vi "RTS Extract Door Test Array.vi"(8 "error in (no error)":errorcluster, 9 "Section Name":string, 10 "section names":string[](array[string]), 11 "Refnum in":T4) -> (0 "error out":errorcluster, 2 "Array":T1[](array[typedef]) {"Start Time" format="%<%X\n%x>T"; "End Time" format="%<%X\n%x>T"}, 3 "Refnum out":T4, 4 "key names":string[][](array[string]))   [LabVIEW 2016]
uses:
  Type Definitions/RTS Door Ops Client.ctl
  Type Definitions/RTS Door Opening Schedule.ctl
  Type Definitions/RTS Door Ops Sequence.ctl
  <vilib>/Utility/config.llb/Config Data RefNum.ctl
  <vilib>/Utility/config.llb/Read Key (Double).vi
  <vilib>/Utility/config.llb/Read Key (Boolean).vi
  <vilib>/Utility/config.llb/Read Key (U32).vi
  <vilib>/Utility/config.llb/NI_LVConfig.lvlib
panel:
  out "Array 2":T1[](array[typedef]) {"Start Time" format="%<%X\n%x>T"; "End Time" format="%<%X\n%x>T"}
  # "Chamber Conditions:"
  # "Chamber Conditions:"
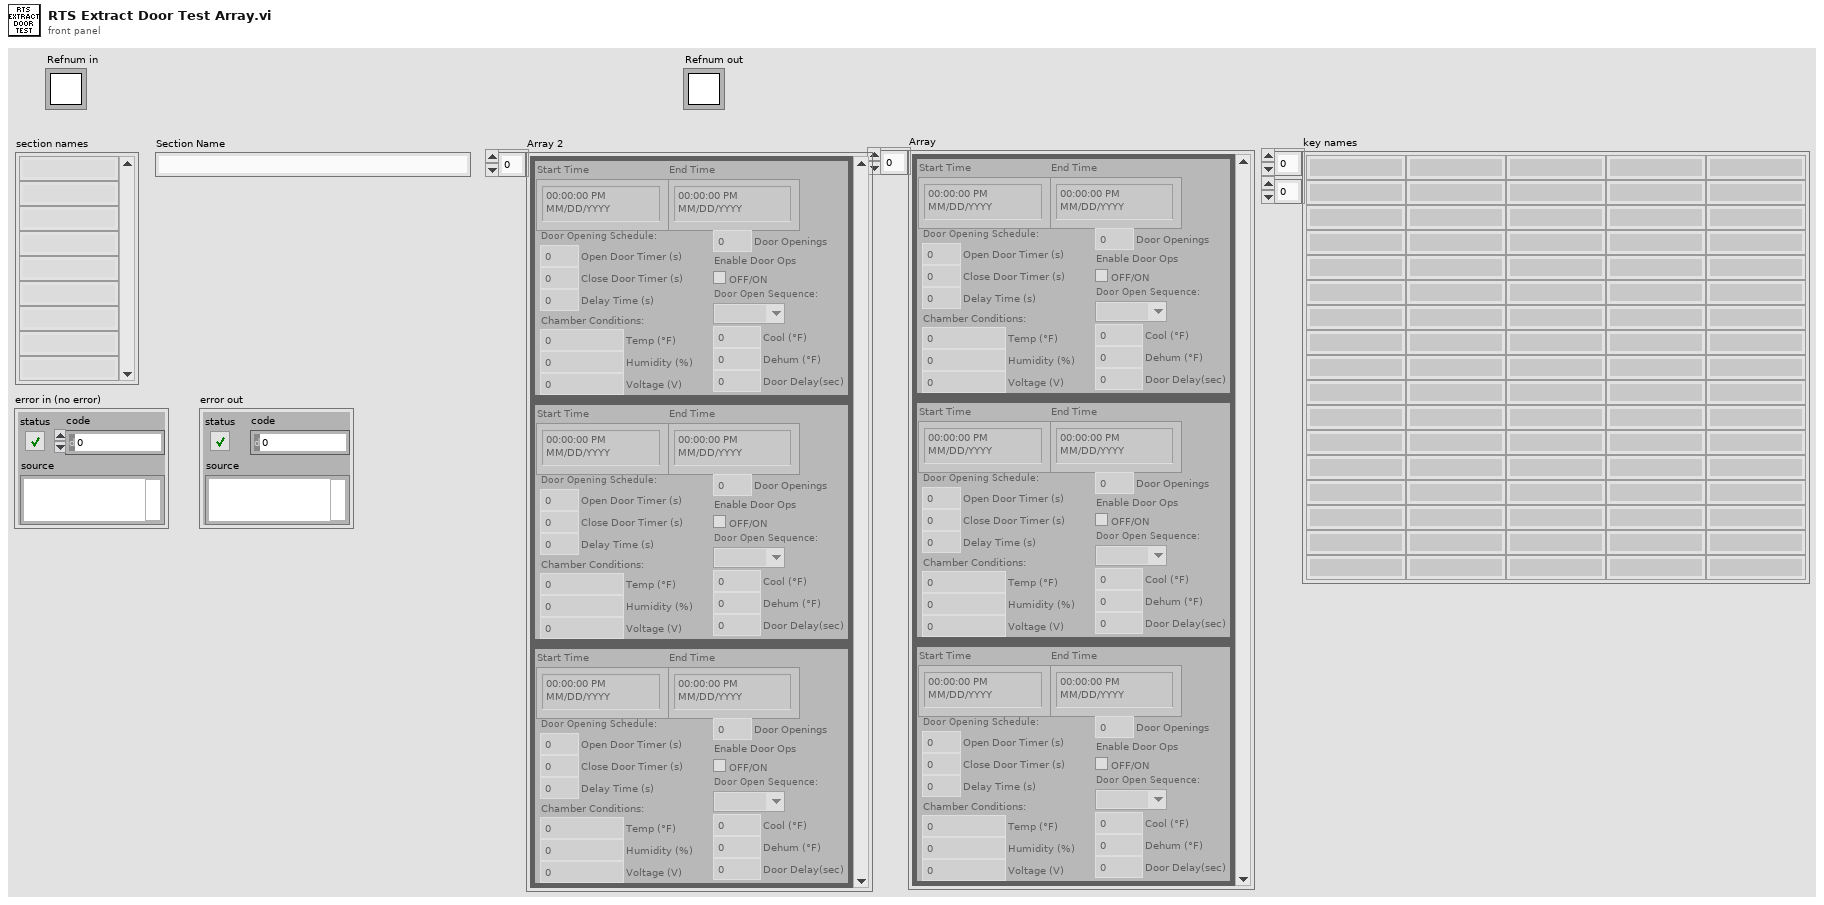
[diagram p1: front panel]
types:
  T1 = typedef "RTS Door Ops Client.ctl" = cluster{"End Time":timestamp, "Start Time":timestamp, "Door Opening Schedule:":T2, "Enable Door Ops":bool, "Door Openings":u32, "Temp (°F)":dbl, "Humidity (%)":dbl, "Voltage (V)":dbl, "Door Open Sequence:":T3, "Door Delay(sec)":dbl, "Dehum (°F)":dbl, "Cool (°F)":dbl}
  T2 = typedef "RTS Door Opening Schedule.ctl" = cluster{"Open Door Timer (s)":dbl, "Delay Time (s)":dbl, "Close Door Timer (s)":dbl}
  T3 = typedef "RTS Door Ops Sequence.ctl" = enum16{"", "1st", "2nd", "3rd"}
  T4 = typedef "NI_LVConfig.lvlib/Config Data RefNum.ctl" = refnum<k1>
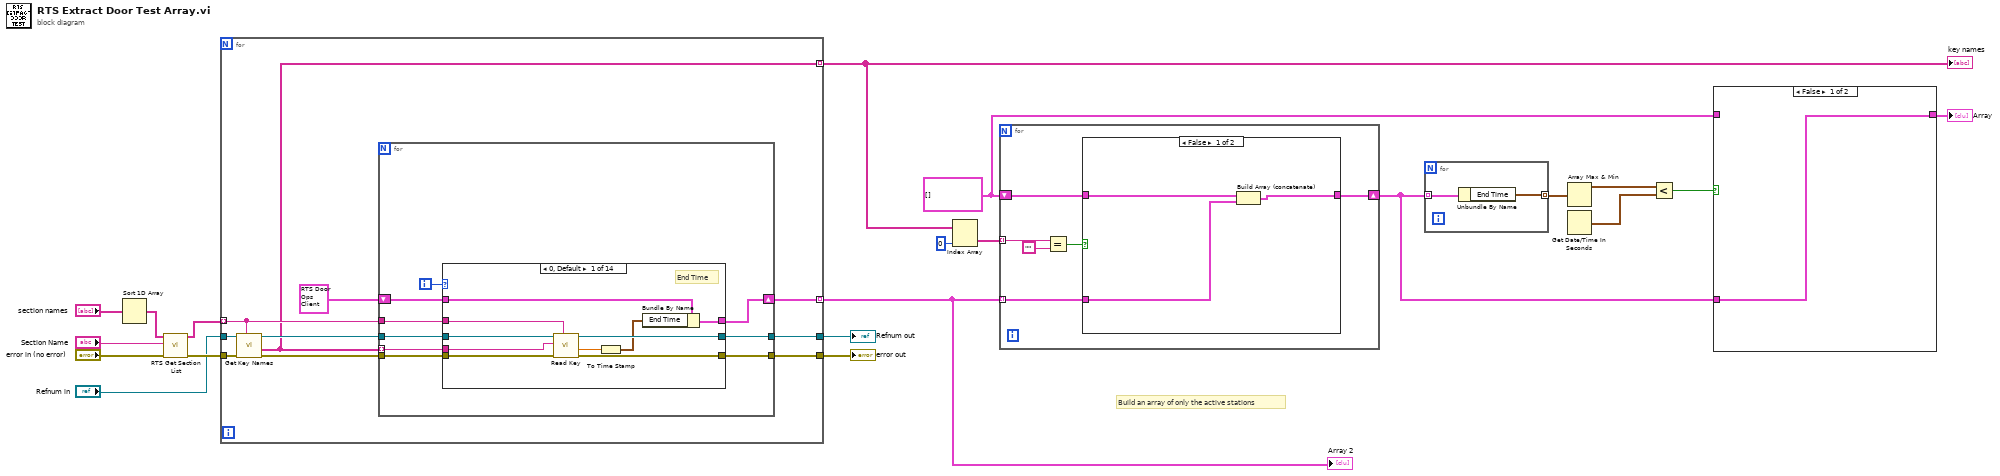
[diagram p0: block diagram]
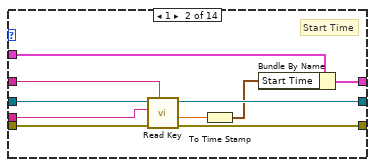
[diagram p4: hidden frame]
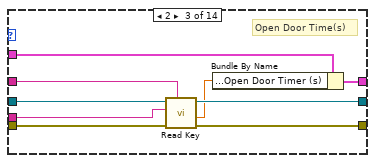
[diagram p5: hidden frame]
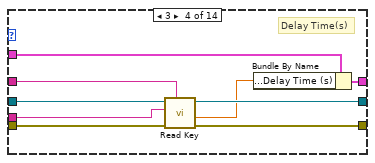
[diagram p6: hidden frame]
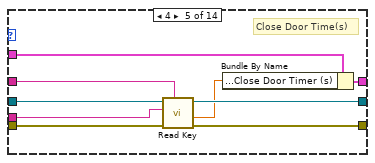
[diagram p7: hidden frame]
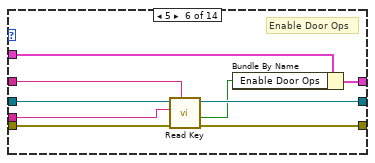
[diagram p8: hidden frame]
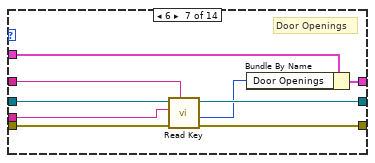
[diagram p9: hidden frame]
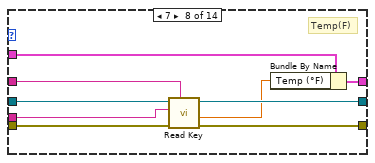
[diagram p10: hidden frame]
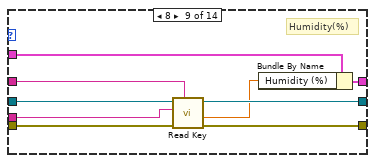
[diagram p11: hidden frame]
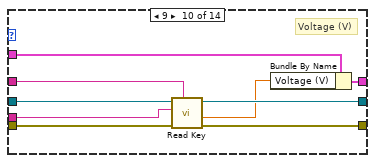
[diagram p12: hidden frame]
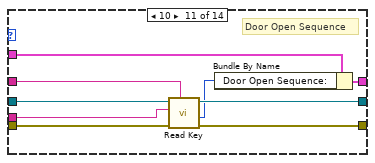
[diagram p13: hidden frame]
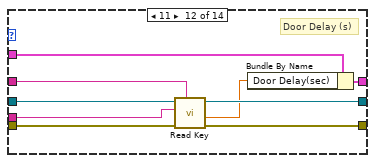
[diagram p14: hidden frame]
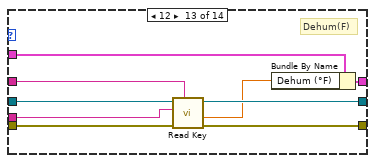
[diagram p15: hidden frame]
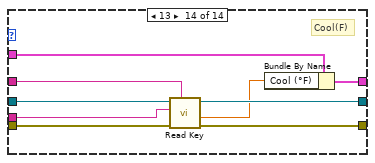
[diagram p16: hidden frame]
diagram:
  w3 = T1[] []
  # "Build an array of only the active stations"
  n1 = Sort 1D Array(array="section names") -> (sorted array=w14:string[])
  n2 = call "RTS Get Section List.vi"("Error In"="error in (no error)", "Section Name"="Section Name", "Sorted Array"=w14) -> ("Error Out"=w20:errorcluster, "Parsed Array"=w17:string[])  [unwired: 7 in]
  n3 = for {
    tunnel: w17 -> [w24] mode=indexing
    tunnel: [w30] -> w8 mode=indexing
    tunnel: "Refnum in" -> [w29]
    tunnel: [w23] -> w15
    tunnel: w20 -> [w28]
    tunnel: [w22] -> w16
    tunnel: [w21] -> w11 mode=indexing
    n4 = call <vilib>:"Get Key Names.vi"("section"=w24, "error in (no error)"=w28, "refnum"=w29) -> ("error out"=w27:errorcluster, "key names"=w21:string[], "refnum out"=w26:T4)  [unwired: 5 in, 1 out]
    n5 = for {
      tunnel: w21 -> [w35] mode=indexing
      shift-right: [w33] -> w30
      shift-left: T1 {"End Time"=timestamp(0 s since 1904-01-01), "Start Time"=timestamp(0 s since 1904-01-01), "Door Opening Schedule:"={"Open Door Timer (s)"=0.0, "Delay Time (s)"=0.0, "Close Door Timer (s)"=0.0}, "Enable Door Ops"=FALSE, "Door Openings"=0, "Temp (°F)"=0.0, "Humidity (%)"=0.0, "Voltage (V)"=0.0, "Door Open Sequence:"=enum."", "Door Delay(sec)"=0.0, "Dehum (°F)"=0.0, "Cool (°F)"=0.0} ("element") -> [w34]
      tunnel: w24 -> [w32]
      tunnel: w26 -> [w36]
      tunnel: [w37] -> w23
      tunnel: w27 -> [w39]
      tunnel: [w38] -> w22
      i -> [w31]
      n6 = case shown="0, Default" w31 {
        tunnel: w39 -> [w48 w58 w68 w76 w86 w94 w103 w112 w121 w130 w139 w148 w157 w167]
        tunnel: [w46 w57 w67 w75 w85 w93 w102 w111 w120 w129 w138 w147 w156 w166] -> w38
        tunnel: [w47 w56 w66 w74 w83 w92 w101 w110 w119 w128 w137 w146 w155 w165] -> w37
        tunnel: w36 -> [w49 w59 w65 w77 w84 w95 w104 w113 w122 w131 w140 w149 w158 w164]
        tunnel: w35 -> [w45 w54 w63 w72 w81 w90 w99 w108 w117 w126 w135 w144 w154 w162]
        tunnel: w34 -> [w43 w52 w62 w71 w80 w89 w98 w107 w116 w125 w134 w143 w152 w161]
        tunnel: [w42 w51 w61 w70 w79 w88 w97 w106 w115 w124 w133 w142 w151 w160] -> w33
        tunnel: w32 -> [w44 w55 w64 w73 w82 w91 w100 w109 w118 w127 w136 w145 w153 w163]
        frame 0, Default {
          # "End Time"
          n7 = call-poly <vilib>:"Read Key.vi"("section"=w44, "error in (no error)"=w48, "key"=w45, "refnum"=w49) -> ("error out"=w46:errorcluster, "value"=w41:dbl, "refnum out"=w47:T4)  [unwired: 4 in, 1 out]
          n8 = To Time Stamp(1:w41) -> (0:w40:timestamp)
          n9 = Bundle By Name(cluster=w43, "End Time"=w40) -> (w42:T1)
        }
        frame 1 {
          # "Start Time"
          n10 = call-poly <vilib>:"Read Key.vi"("section"=w55, "error in (no error)"=w58, "key"=w54, "refnum"=w59) -> ("error out"=w57:errorcluster, "value"=w53:dbl, "refnum out"=w56:T4)  [unwired: 4 in, 1 out]
          n11 = To Time Stamp(1:w53) -> (0:w50:timestamp)
          n12 = Bundle By Name(cluster=w52, "Start Time"=w50) -> (w51:T1)
        }
        frame 2 {
          # "Open Door Time(s)"
          n13 = call-poly <vilib>:"Read Key.vi"("section"=w64, "error in (no error)"=w68, "key"=w63, "refnum"=w65) -> ("error out"=w67:errorcluster, "value"=w60:dbl, "refnum out"=w66:T4)  [unwired: 4 in, 1 out]
          n14 = Bundle By Name(cluster=w62, "Door Opening Schedule:.Open Door Timer (s)"=w60) -> (w61:T1)
        }
        frame 3 {
          # "Delay Time(s)"
          n15 = call-poly <vilib>:"Read Key.vi"("section"=w73, "error in (no error)"=w76, "key"=w72, "refnum"=w77) -> ("error out"=w75:errorcluster, "value"=w69:dbl, "refnum out"=w74:T4)  [unwired: 4 in, 1 out]
          n16 = Bundle By Name(cluster=w71, "Door Opening Schedule:.Delay Time (s)"=w69) -> (w70:T1)
        }
        frame 4 {
          # "Close Door Time(s)"
          n17 = call-poly <vilib>:"Read Key.vi"("section"=w82, "error in (no error)"=w86, "key"=w81, "refnum"=w84) -> ("error out"=w85:errorcluster, "value"=w78:dbl, "refnum out"=w83:T4)  [unwired: 4 in, 1 out]
          n18 = Bundle By Name(cluster=w80, "Door Opening Schedule:.Close Door Timer (s)"=w78) -> (w79:T1)
        }
        frame 5 {
          # "Enable Door Ops"
          n19 = call-poly <vilib>:"Read Key.vi"("section"=w91, "error in (no error)"=w94, "key"=w90, "refnum"=w95) -> ("error out"=w93:errorcluster, "value"=w87:bool, "refnum out"=w92:T4)  [unwired: 4 in, 1 out]
          n20 = Bundle By Name(cluster=w89, "Enable Door Ops"=w87) -> (w88:T1)
        }
        frame 6 {
          # "Door Openings"
          n21 = call-poly <vilib>:"Read Key.vi"("section"=w100, "error in (no error)"=w103, "key"=w99, "refnum"=w104) -> ("error out"=w102:errorcluster, "value"=w96:u32, "refnum out"=w101:T4)  [unwired: 4 in, 1 out]
          n22 = Bundle By Name(cluster=w98, "Door Openings"=w96) -> (w97:T1)
        }
        frame 7 {
          # "Temp(F)"
          n23 = call-poly <vilib>:"Read Key.vi"("section"=w109, "error in (no error)"=w112, "key"=w108, "refnum"=w113) -> ("error out"=w111:errorcluster, "value"=w105:dbl, "refnum out"=w110:T4)  [unwired: 4 in, 1 out]
          n24 = Bundle By Name(cluster=w107, "Temp (°F)"=w105) -> (w106:T1)
        }
        frame 8 {
          # "Humidity(%)"
          n25 = call-poly <vilib>:"Read Key.vi"("section"=w118, "error in (no error)"=w121, "key"=w117, "refnum"=w122) -> ("error out"=w120:errorcluster, "value"=w114:dbl, "refnum out"=w119:T4)  [unwired: 4 in, 1 out]
          n26 = Bundle By Name(cluster=w116, "Humidity (%)"=w114) -> (w115:T1)
        }
        frame 9 {
          # "Voltage (V)"
          n27 = call-poly <vilib>:"Read Key.vi"("section"=w127, "error in (no error)"=w130, "key"=w126, "refnum"=w131) -> ("error out"=w129:errorcluster, "value"=w123:dbl, "refnum out"=w128:T4)  [unwired: 4 in, 1 out]
          n28 = Bundle By Name(cluster=w125, "Voltage (V)"=w123) -> (w124:T1)
        }
        frame 10 {
          # "Door Open Sequence"
          n29 = call-poly <vilib>:"Read Key.vi"("section"=w136, "error in (no error)"=w139, "key"=w135, "refnum"=w140) -> ("error out"=w138:errorcluster, "value"=w132:u32, "refnum out"=w137:T4)  [unwired: 4 in, 1 out]
          n30 = Bundle By Name(cluster=w134, "Door Open Sequence:"=w132) -> (w133:T1)
        }
        frame 11 {
          # "Door Delay (s)"
          n31 = call-poly <vilib>:"Read Key.vi"("section"=w145, "error in (no error)"=w148, "key"=w144, "refnum"=w149) -> ("error out"=w147:errorcluster, "value"=w141:dbl, "refnum out"=w146:T4)  [unwired: 4 in, 1 out]
          n32 = Bundle By Name(cluster=w143, "Door Delay(sec)"=w141) -> (w142:T1)
        }
        frame 12 {
          # "Dehum(F)"
          n33 = call-poly <vilib>:"Read Key.vi"("section"=w153, "error in (no error)"=w157, "key"=w154, "refnum"=w158) -> ("error out"=w156:errorcluster, "value"=w150:dbl, "refnum out"=w155:T4)  [unwired: 4 in, 1 out]
          n34 = Bundle By Name(cluster=w152, "Dehum (°F)"=w150) -> (w151:T1)
        }
        frame 13 {
          # "Cool(F)"
          n35 = call-poly <vilib>:"Read Key.vi"("section"=w163, "error in (no error)"=w167, "key"=w162, "refnum"=w164) -> ("error out"=w166:errorcluster, "value"=w159:dbl, "refnum out"=w165:T4)  [unwired: 4 in, 1 out]
          n36 = Bundle By Name(cluster=w161, "Cool (°F)"=w159) -> (w160:T1)
        }
      }
    }
  }
  "error out" <- w16
  "Refnum out" <- w15
  "key names" <- w11
  "Array 2" <- w8
  n37 = Index Array(array=w11, index (col)=0 ("disabled index (col)")) -> (element=w9:string[])  [unwired: 1 in]
  n38 = for {
    tunnel: w9 -> [w173] mode=indexing
    shift-right: [w169] -> w1
    shift-left: w3 -> [w170]
    tunnel: w8 -> [w168] mode=indexing
    n39 = Equal?(x=w173, y="") -> (x = y?=w171:bool)
    n40 = case shown="False" w171 {
      tunnel: w170 -> [w176 w177]
      tunnel: [w175 w177] -> w169
      tunnel: w168 -> [w174 _]
      frame False {
        n41 = Build Array (concatenate)(w176, w174) -> (w175:T1[])
      }
      frame True {
      }
    }
  }
  n42 = for {
    tunnel: w1 -> [w179] mode=indexing
    tunnel: [w178] -> w7 mode=indexing
    n43 = Unbundle By Name(w179) -> ("End Time"=w178:timestamp)
  }
  n44 = Array Max & Min(array=w7) -> (max value=w6:timestamp)  [unwired: 3 out]
  n45 = Get Date/Time In Seconds() -> (seconds since 1Jan1904=w5:timestamp)
  n46 = Less?(x=w6, y=w5) -> (x < y?=w4:bool)
  n47 = case shown="False" w4 {
    tunnel: w3 -> [_ w181]
    tunnel: [w180 w181] -> w2
    tunnel: w1 -> [w180 _]
    frame False {
    }
    frame True {
    }
  }
  "Array" <- w2
